vi "Read Resistor.vi"() -> (0 "Resistance":T1=enum."1G ohm")   [LabVIEW 2019, in "Relay-Box.lvclass"]
uses:
  Relay-Box.lvclass
  Typedefs/Resistor--enum.ctl
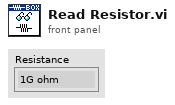
[diagram p1: front panel]
types:
  T1 = typedef "Relay-Box.lvclass/Resistor--enum.ctl" = enum16{"open", "discharge tip", "0 ohms", "100k ohm", "10M ohm", "1G ohm"}
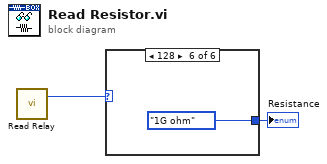
[diagram p0: block diagram]
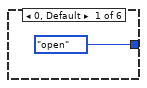
[diagram p2: hidden frame]
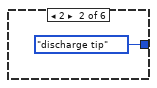
[diagram p3: hidden frame]
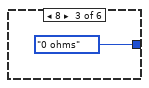
[diagram p4: hidden frame]
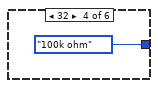
[diagram p5: hidden frame]
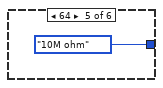
[diagram p6: hidden frame]
diagram:
  n1 = call "Read Relay.vi"() -> ("unsigned 8bit integer"=w2:u8)  [unwired: 1 in, 1 out]
  n2 = case shown="128" w2 {
    tunnel: [Resistor--enum."open" ("Set Resistance") Resistor--enum."discharge tip" ("Set Resistance") Resistor--enum."0 ohms" ("Set Resistance") Resistor--enum."100k ohm" ("Set Resistance") Resistor--enum."10M ohm" ("Set Resistance") Resistor--enum."1G ohm" ("Set Resistance")] -> w1
    frame 0, Default {
    }
    frame 2 {
    }
    frame 8 {
    }
    frame 32 {
    }
    frame 64 {
    }
    frame 128 {
    }
  }
  "Resistance" <- w1
